vi "Timer Dialog.vi"(8 "error in (no error)":errorcluster, 10 "Timeout":dbl=5.0, 11 "Message In":string="PLEASE WAIT FOR 5 MINS...") -> (0 "error out":errorcluster, 3 "Selection":bool)   [LabVIEW 2020]
doc: "Selection is true if Yes was pressed or on timeout. Selection is false only if No was pressed before timeout."
panel:
  in  "No":bool
  in  "Yes":bool
  out "Message":string
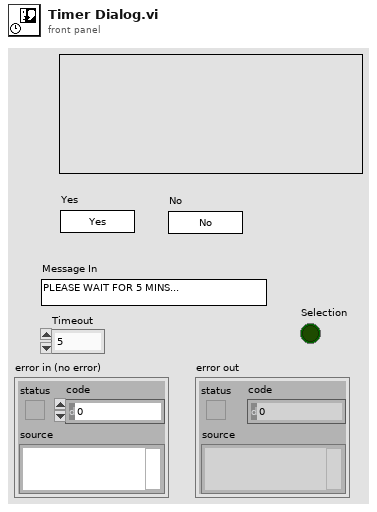
[diagram p1: front panel]
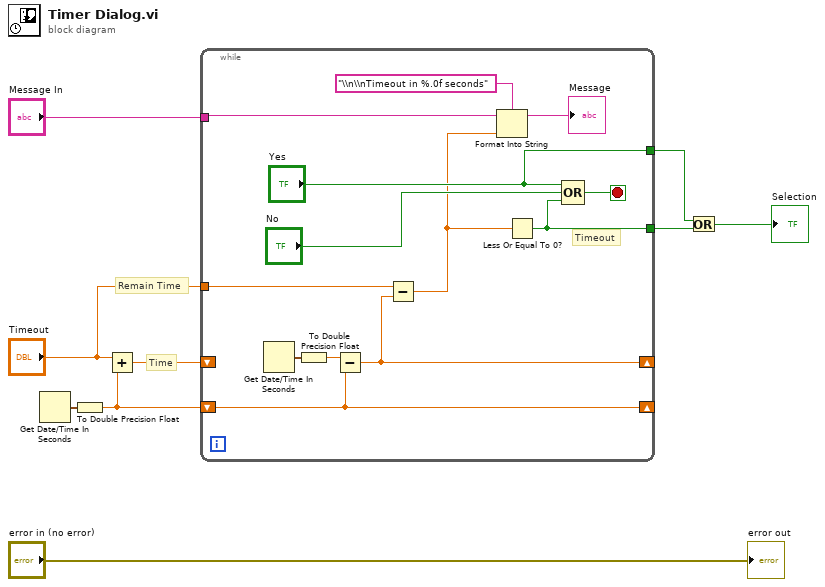
[diagram p0: block diagram]
diagram:
  # "Time"
  # "Remain Time"
  n1 = Get Date/Time In Seconds() -> (seconds since 1Jan1904=w8:timestamp)
  n2 = To Double Precision Float(number=w8) -> (double precision float=w6:dbl)
  n3 = Add(x="Timeout", y=w6) -> (x+y=w7:dbl)
  n4 = while {
    shift-right: [w18] -> _
    shift-left: w7 -> [_]
    shift-right: [w20] -> _
    shift-left: w6 -> [w20]
    tunnel: "Timeout" -> [w19]
    tunnel: [w16] -> w4
    tunnel: ["Yes"] -> w3
    tunnel: "Message In" -> [w13]
    stop <- w17 stop-if-true
    # "Timeout"
    n5 = Get Date/Time In Seconds() -> (seconds since 1Jan1904=w22:timestamp)
    n6 = To Double Precision Float(number=w22) -> (double precision float=w21:dbl)
    n7 = Subtract(x=w21, y=w20) -> (x-y=w18:dbl)
    n8 = Subtract(x=w19, y=w18) -> (x-y=w12:dbl)
    n9 = Format Into String(format string="\\n\\nTimeout in %.0f seconds", initial string=w13, w12) -> (resulting string=→"Message":string)  [unwired: 1 in, 1 out]
    n10 = Less Or Equal To 0?(x=w12) -> (x <= 0?=w16:bool)
    n11 = Compound Arithmetic op=OR("Yes", "No", w16) -> (w17:bool)
  }
  n12 = Or(x=w3, y=w4) -> (x .or. y?=→"Selection":bool)
  "error out" <- "error in (no error)"
